vi "Add data to db generic.vi"() -> ()   [LabVIEW 2014]
uses:
  <vilib>/addons/database/Connection.llb/DB Tools Open Connec (Path).vi
  <vilib>/addons/database/NI_Database_API.lvlib
panel:
  out "data":string[][](table)
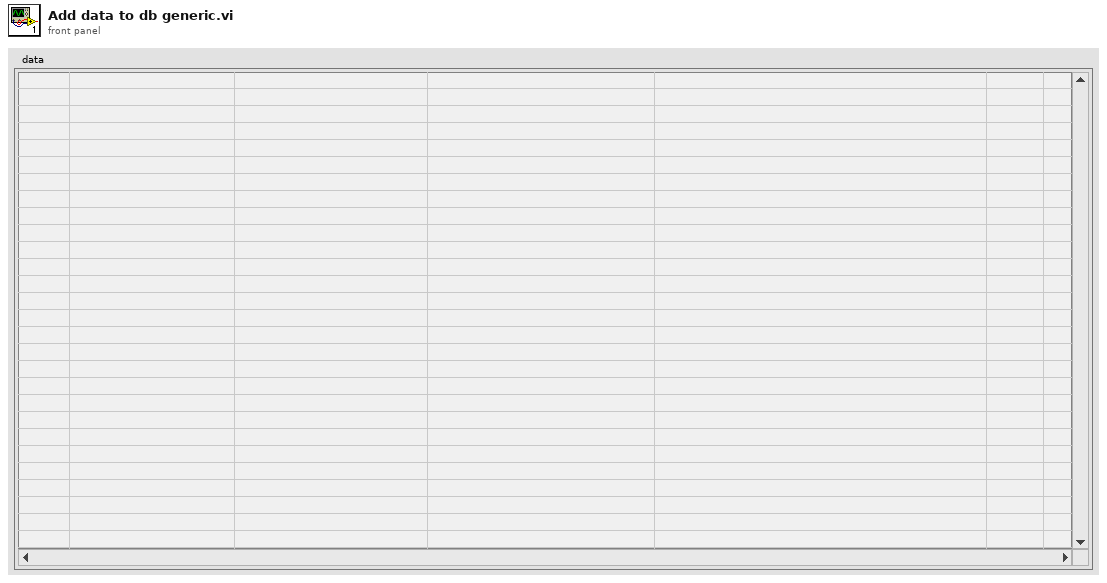
[diagram p1: front panel]
types:
  T1 = typedef "NI_Database_API.lvlib/Conn ObjectReference.ctl" = refnum<k1>
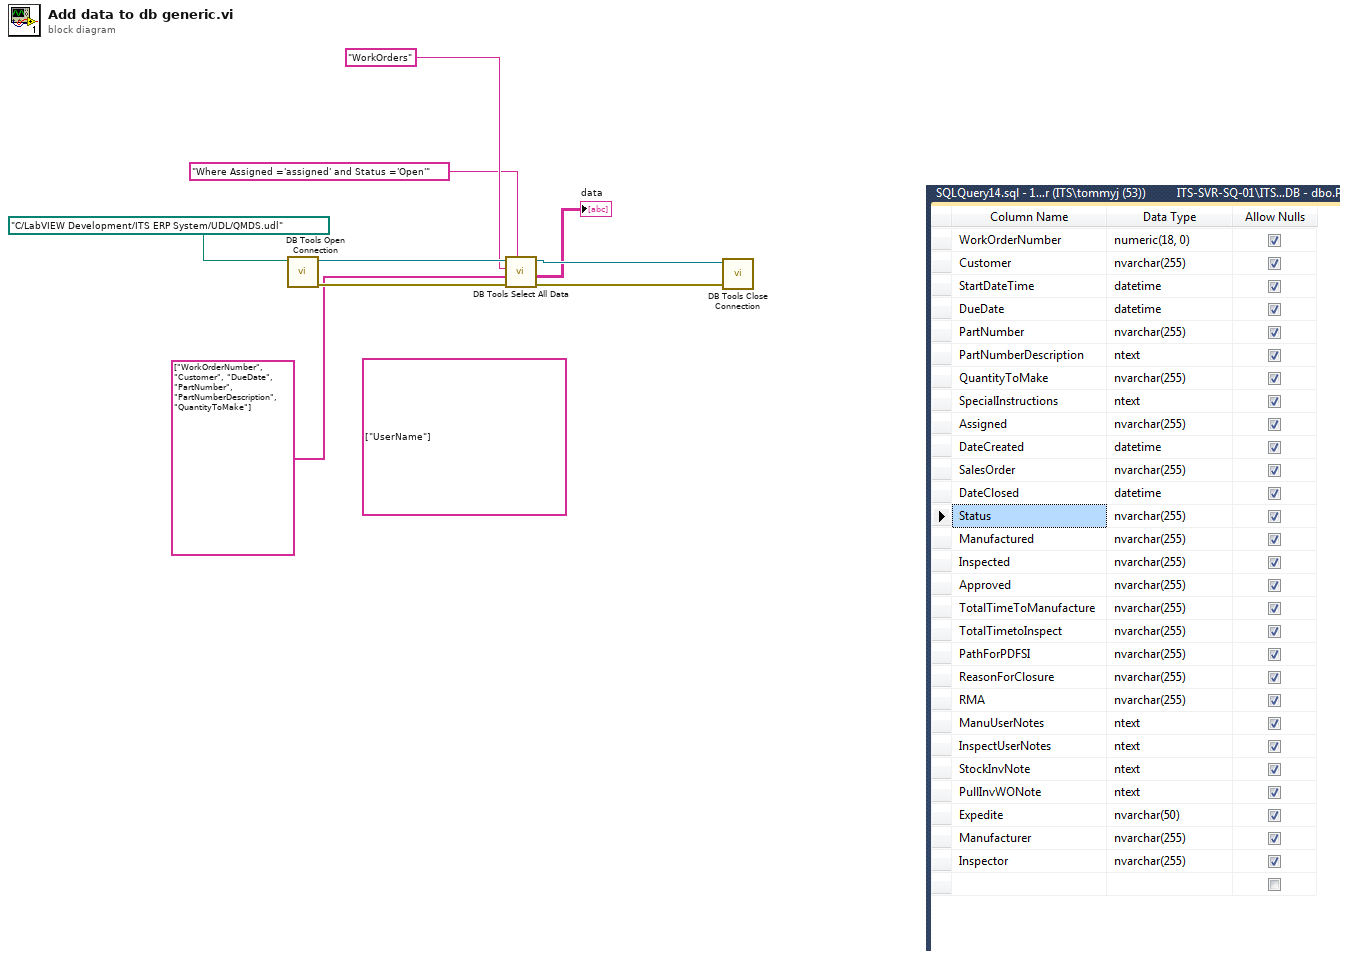
[diagram p0: block diagram]
diagram:
  (unwired) string[] ["UserName"] ("columns")
  n1 = call-poly <vilib>:"DB Tools Open Connection.vi"("connection information"=path "C:/LabVIEW Development/ITS ERP System/UDL/QMDS.udl" ("Database (mdb)  File Path")) -> ("error out"=w7:errorcluster, "connection reference"=w8:T1)  [unwired: 7 in]
  n2 = call <vilib>:"DB Tools Select All Data.vi"("optional clause"="Where Assigned ='assigned' and Status ='Open'", "error in (no error)"=w7, "columns"=string[] ["WorkOrderNumber", "Customer", "DueDate", "PartNumber", "PartNumberDescription", "QuantityToMake"], "table"="WorkOrders" ("Table"), "connection reference"=w8) -> ("error out"=w3:errorcluster, "data"=→"data":string[][], "connection reference out"=w4:T1)  [unwired: 1 in]
  n3 = call <vilib>:"DB Tools Close Connection.vi"("error in (no error)"=w3, "connection reference"=w4) -> ()  [unwired: 5 in, 1 out]
